vi "ADQ214 Get Ptr Data Ch B.vi"(8 "error in (no error)":errorcluster, 10 "adq214_num":i32, 11 "adq_cu_ptr":u32) -> (0 "error out":errorcluster, 2 "function return":i32, 3 "adq_cu_ptr out":u32)   [LabVIEW 2009, in "ADQAPI.lvlib"]
doc: "extern \"C\" __declspec(dllimport) int* ADQ214_GetPtrDataChB(void* adq_cu_ptr, int adq214_num);"
uses:
  ADQAPI.lvlib
  ADQAPI.dll
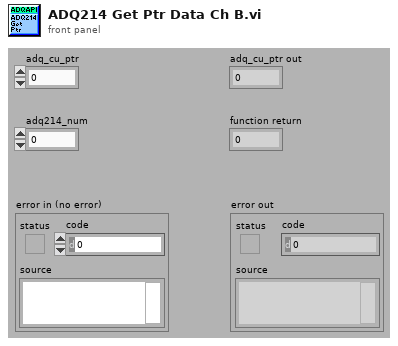
[diagram p1: front panel]
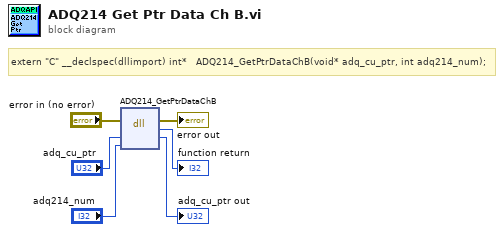
[diagram p0: block diagram]
diagram:
  # "extern \"C\" __declspec(dllimport) int*\t\t\tADQ214_GetPtrDataChB(void* adq_cu_ptr, int adq214_num);"
  n1 = dll-call lib="ADQAPI.*" fn="ADQ214_GetPtrDataChB"(error in="error in (no error)", "adq_cu_ptr"="adq_cu_ptr", "adq214_num"="adq214_num") -> (error out=→"error out":errorcluster, →"function return":i32, "adq_cu_ptr"=→"adq_cu_ptr out":u32)  [unwired: 3 in, 1 out]
